vi "coordinates_to_distance.vi"(8 "end lon":dbl, 9 "end lat":dbl, 10 "start lon":dbl, 11 "start lat":dbl) -> (3 "distance [m]":dbl)   [LabVIEW 2019]
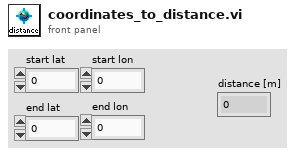
[diagram p1: front panel]
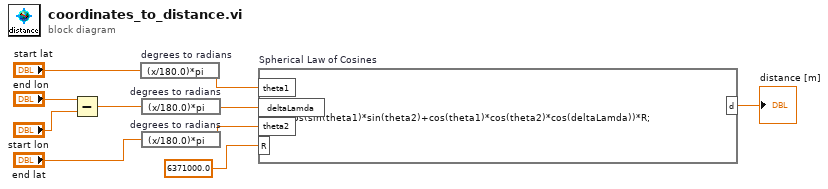
[diagram p0: block diagram]
diagram:
  n1 = Subtract(x="end lon", y="start lon") -> (x-y=w10:dbl)
  n2 = expression code="(x/180.0)*pi" "degrees to radians"("start lat") -> (w8:dbl)
  n3 = expression code="(x/180.0)*pi" "degrees to radians"(w10) -> (w9:dbl)
  n4 = expression code="(x/180.0)*pi" "degrees to radians"("end lat") -> (w7:dbl)
  n5 = formula code="d=acos(sin(theta1)*sin(theta2)+cos(theta1)*cos(theta2)*cos(deltaLamda))*R;" "Spherical Law of Cosines"("theta1"=w8, "theta2"=w7, "deltaLamda"=w9, "R"=6371000.0 ("input variable")) -> ("d"=→"distance [m]":dbl)
